vi "Escape String Tree.vi"(9 "Reverse? (False)":bool, 10 "Escapes":cluster{"String":string, "Escape":string}[](array[cluster]), 11 "String In":string) -> (3 "String Out":string)   [LabVIEW 2020, in "NI_VIAnCFGDataStructure.lvlib" / "Tree.lvclass"]
doc: "Adds or Removes escapes to or from a string.\n\n<B>String In</B> - The string to handle escapes in,\n<B>Escapes</B> - The escape patterns to handle. When adding escapes, they are added in the order of the array. If removing escapes, they are removed in reverse order.\n<B>Reverse?</B> - Should the escapes be added or removed.\n<B>String Out</B> - The resulting string with the escapes handled."
uses:
  <vilib>/addons/analyzer/VIAnCFGDataStructure/Tree Manager/Tree.lvclass
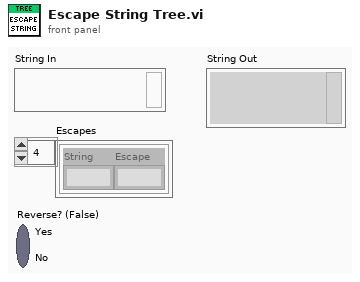
[diagram p1: front panel]
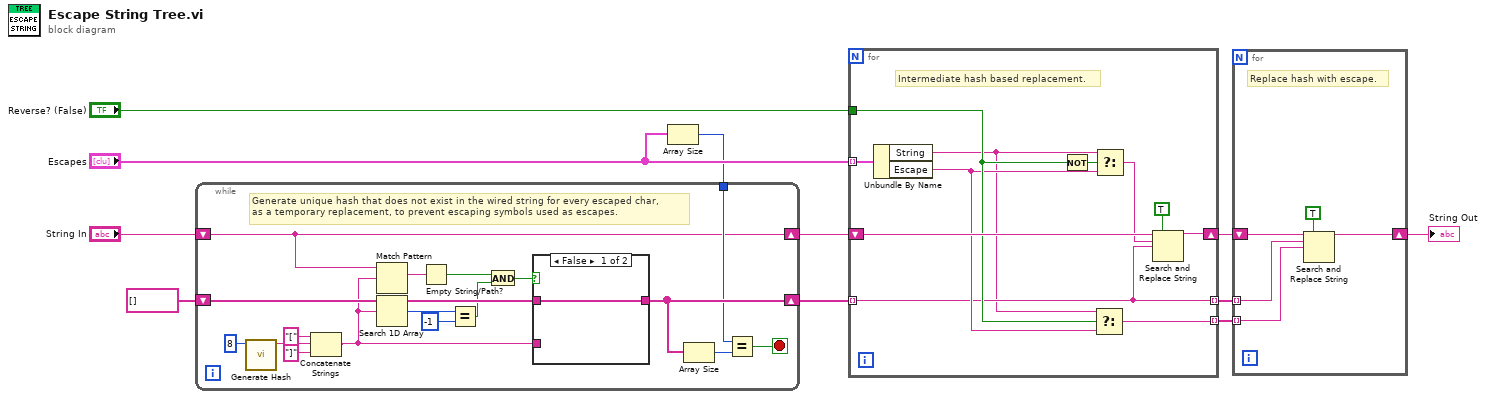
[diagram p0: block diagram]
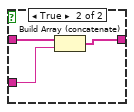
[diagram p2: hidden frame]
diagram:
  n1 = Array Size(array="Escapes") -> (size(s)=w4:i32)
  n2 = while {
    shift-right: [w26] -> w3
    shift-left: string[] [] -> [w27]
    tunnel: w4 -> [w23]
    shift-right: [w12] -> w1
    shift-left: "String In" -> [w12]
    stop <- w24 stop-if-true
    # "Generate unique hash that does not exist in the wired string for every escaped char,\nas a temporary replacement, to prevent escaping symbols used as escapes."
    n3 = call <vilib>:"Generate Hash.vi"("Size (16)"=8) -> ("Hash"=w20:string)  [unwired: 9 in, 1 out]
    n4 = Concatenate Strings("[" ("string"), w20, "]" ("string")) -> (w19:string)
    n5 = Match Pattern(string=w12, regular expression=w19) -> (match substring=w16:string)  [unwired: 1 in, 3 out]
    n6 = Search 1D Array(1D array=w27, element=w19) -> (index of element=w18:i32)  [unwired: 1 in]
    n7 = Empty String/Path?(string/path=w16) -> (empty?=w14:bool)
    n8 = Equal?(x=w18, y=-1) -> (x = y?=w15:bool)
    n9 = And(x=w14, y=w15) -> (x .and. y?=w13:bool)
    n10 = case shown="False" w13 {
      tunnel: w19 -> [_ w32]
      tunnel: [w29 w31] -> w26
      tunnel: w27 -> [w29 w30]
      frame False {
      }
      frame True {
        n11 = Build Array (concatenate)(w30, w32) -> (w31:string[])
      }
    }
    n12 = Array Size(array=w26) -> (size(s)=w25:i32)
    n13 = Equal?(x=w23, y=w25) -> (x = y?=w24:bool)
  }
  n14 = for {
    tunnel: "Escapes" -> [w43] mode=indexing
    shift-right: [w40] -> w10
    shift-left: w1 -> [w41]
    tunnel: [w34] -> w9 mode=indexing
    tunnel: [w35] -> w8 mode=indexing
    tunnel: "Reverse? (False)" -> [w37]
    tunnel: w3 -> [w34] mode=indexing
    # "Intermediate hash based replacement."
    n15 = Unbundle By Name(w43) -> ("String"=w33:string, "Escape"=w36:string)
    n16 = Not(x=w37) -> (.not. x?=w39:bool)
    n17 = Select(t=w33, s=w37, f=w36) -> (s? t:f=w35:string)
    n18 = Select(t=w33, s=w39, f=w36) -> (s? t:f=w38:string)
    n19 = Search and Replace String(replace all?=TRUE ("replace all? (F)"), input string=w41, search string=w38, replace string=w34) -> (result string=w40:string)  [unwired: 4 in, 3 out]
  }
  n20 = for {
    shift-right: [w46] -> w11
    shift-left: w10 -> [w48]
    tunnel: w9 -> [w45] mode=indexing
    tunnel: w8 -> [w44] mode=indexing
    # "Replace hash with escape."
    n21 = Search and Replace String(replace all?=TRUE ("replace all? (F)"), input string=w48, search string=w45, replace string=w44) -> (result string=w46:string)  [unwired: 4 in, 3 out]
  }
  "String Out" <- w11
